vi "Port to Read.vi"(8 "error in (no error)":errorcluster, 10 "Port to Read":dbl, 11 "Arduino in":refnum<class "Arduino.lvclass">) -> (0 "error out":errorcluster, 3 "Arduino out":refnum<class "Arduino.lvclass">)   [LabVIEW 2020, in "Arduino.lvclass"]
doc: "Port to read es el vi donde se manda al microcontrolador los datos del puerto que se desea leer"
uses:
  Arduino.lvclass
  Arduino.lvclass/Arduino.ctl
  b5b80321-8997-40e9-9077-6da0740c4efa.vi
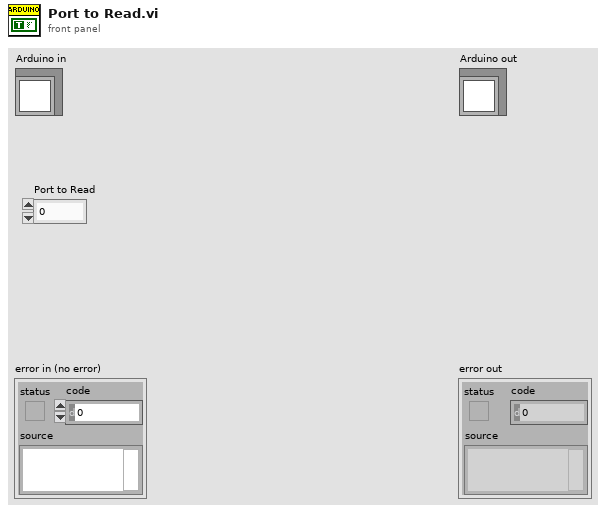
[diagram p1: front panel]
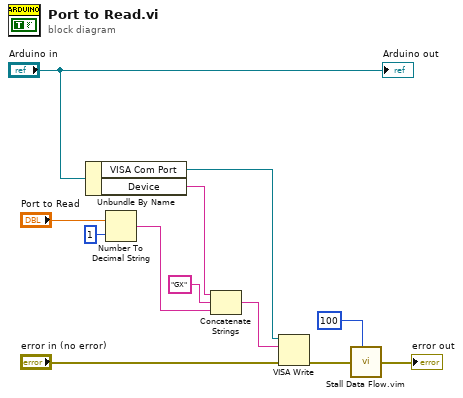
[diagram p0: block diagram]
diagram:
  n1 = Unbundle By Name("Arduino in") -> ("VISA Com Port"=w11:refnum<visa-resource-name>, "Device"=w9:string)
  n2 = Number To Decimal String(number="Port to Read", width (-)=i16 1) -> (decimal integer string=w8:string)
  n3 = Concatenate Strings(w9, "GX" ("string"), w8) -> (w10:string)
  n4 = VISA Write(VISA resource name=w11, write buffer=w10, error in (no error)="error in (no error)") -> (error out=w12:errorcluster)  [unwired: 2 out]
  n5 = call "Stall Data Flow.vim"("value in"=w12, "milliseconds to wait"=u32 100) -> ("value out"=→"error out":errorcluster)  [unwired: 1 out]
  "Arduino out" <- "Arduino in"
